vi "Details Display Dialog.vi"(0 "Source":string, 1 "Start":i32[](array[numeric]), 2 "Length":i32[](array[numeric]), 5 "Details":string="reason for problem", 7 "dialog type":T2, 9 "Error or Warning":bool, 11 "contname":string="Continue", 12 "stopname":string="Stop", 13 "okname":string="OK") -> (15 "stop event propagated":bool)   [LabVIEW 2011]
uses:
  DialogTypeEnum.ctl
  ErrWarn.ctl
  eventvkey.ctl
panel:
  in  "truncated message":string="(source truncated)"
  in  "truncated & CH message":string="(source truncated; see Context Help window)"
  out "Source of Error":string
  out "scrollbar text":string
  in  "Test for size":string
  out "text":string
  out "Error or Warning Glyph":T1=TRUE
  in  "OK":bool
  in  "Stop":bool
  in  "Continue":bool
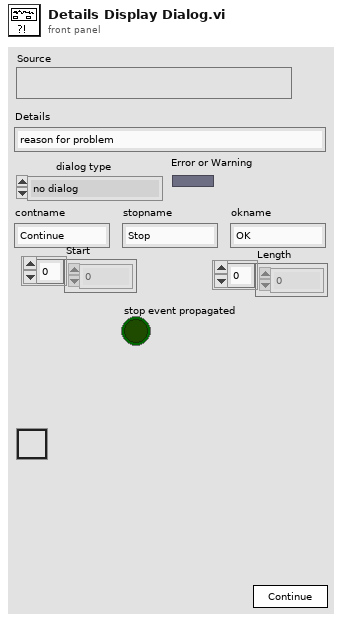
[diagram p1: front panel]
types:
  T1 = typedef "ErrWarn.ctl" = bool
  T2 = typedef "DialogTypeEnum.ctl" = enum16{"no dialog", "OK message", "continue or stop message", "auto error handling dialog", "OK message + warnings", "continue/stop + warnings"}
  T3 = typedef "eventvkey.ctl" = enum16{"ASCII", "Enter", "Return", "Shift", "Ctrl", "Alt", "Cmd", "Opt", "Caps", "NumLock", "Clear", "Break", "Up", "Down", "Left", "Right", "Insert", "Delete", "Home", "End", "PageUp", "PageDown", "Escape", "Help", "Pause", "ScrollLock", "F1", "F2", "F3", "F4", "F5", "F6", "F7", "F8", "F9", "F10", "F11", "F12", "F13", "F14", "F15", "F16", "F17", "F18", "F19", "F20", "F21", "F22", "F23", "F24", "Play", "VolumeUp", "VolumeDown", "Mute", "Two Byte Char"}
  T4 = typedef "LVRectTypeDef.ctl" = cluster{"left":i16, "top":i16, "right":i16, "bottom":i16}
  T5 = cluster{"Control":bool, "Shift":bool, "Key":string}
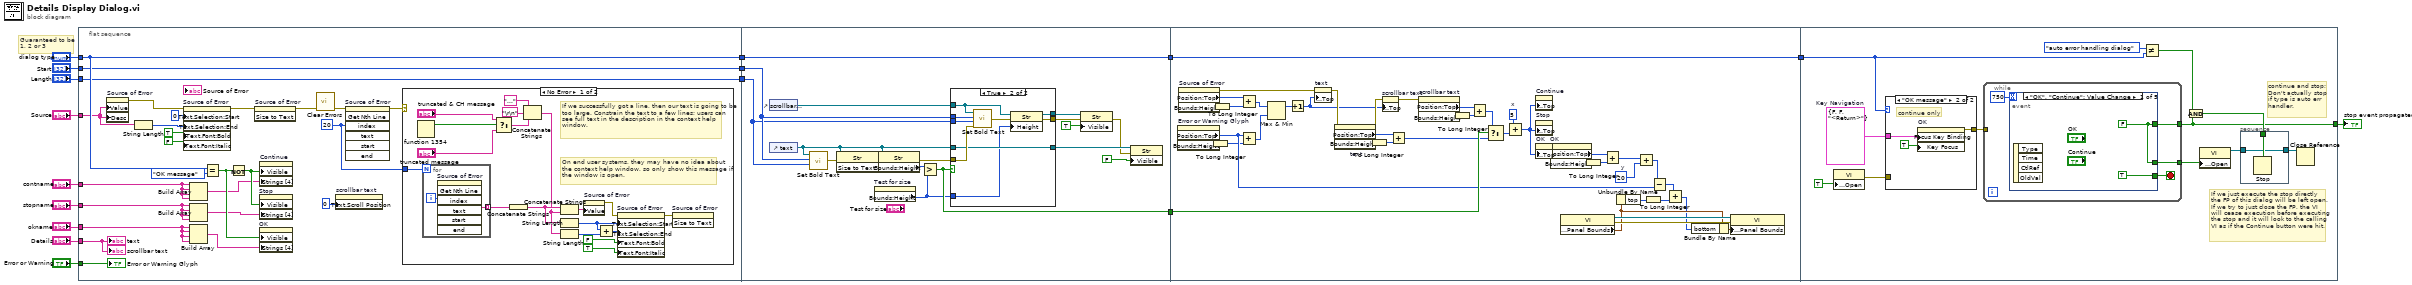
[diagram p0: block diagram]
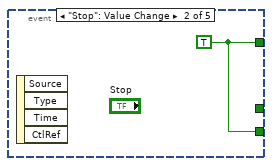
[diagram p4: hidden frame]
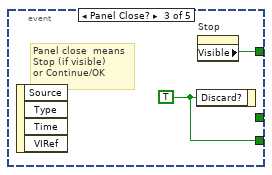
[diagram p5: hidden frame]
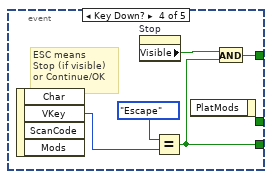
[diagram p6: hidden frame]
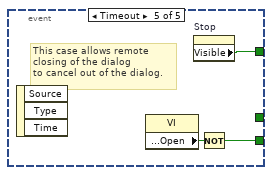
[diagram p7: hidden frame]
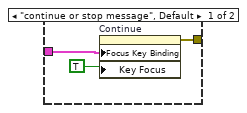
[diagram p8: hidden frame]
diagram:
  # "Guaranteed to be\n1, 2 or 3"
  n1 = flat-sequence {
    tunnel: [w25] -> w15
    tunnel: "dialog type" -> [w25]
    tunnel: "contname" -> [w24]
    tunnel: "stopname" -> [w23]
    tunnel: "okname" -> [w22]
    tunnel: "Source" -> [w17]
    tunnel: "Details" -> [w21]
    tunnel: "Error or Warning" -> [w20]
    tunnel: [w19] -> w4
    tunnel: [w18] -> w3
    tunnel: "Start" -> [w19]
    tunnel: "Length" -> [w18]
    tunnel: w15 -> [w65]
    tunnel: [w65] -> w14
    tunnel: [w71] -> w13
    tunnel: w4 -> [w64]
    tunnel: w3 -> [w63]
    tunnel: w14 -> [w98]
    tunnel: [w98] -> w12
    tunnel: w13 -> [w133]
    tunnel: [w134] -> w16
    tunnel: w12 -> [w136]
    frame #0 {
      w32 = u32 20 ("index")
      n2 = property on="Source of Error" class="Str"("Value"=w17, "Desc"=w17) -> (error out=w31:errorcluster)  [unwired: 2 in, 1 out]
      n3 = String Length(string=w17) -> (length=w28:i32)
      n4 = property on="Source of Error" class="Str"(error in=w31, "Text.Selection:Start"=u32 0, "Text.Selection:End"=w28, "Text.Font:Bold"=TRUE, "Text.Font:Italic"=FALSE) -> (error out=w30:errorcluster)  [unwired: 1 in, 1 out]
      n5 = Build Array(w24, w24, w24, w24) -> (w40:string[])
      n6 = Build Array(w23, w23, w23, w23) -> (w39:string[])
      n7 = Build Array(w22, w22, w22, w22) -> (w38:string[])
      n8 = Equal?(x=w25, y=DialogTypeEnum."OK message" ("dialog type")) -> (x = y?=w42:bool)
      n9 = Not(x=w42) -> (.not. x?=w41:bool)
      n10 = invoke on="Source of Error" class="Str" method="Size to Text"(error in=w30) -> (error out=w35:errorcluster)  [unwired: 2 in, 2 out]
      n11 = property on="Continue" class="Bool"("Visible"=w41, "Strings [4]"=w40) -> ()  [unwired: 2 in, 2 out]
      n12 = property on="Stop" class="Bool"("Visible"=w41, "Strings [4]"=w39) -> ()  [unwired: 2 in, 2 out]
      n13 = property on="OK" class="Bool"("Visible"=w42, "Strings [4]"=w38) -> ()  [unwired: 2 in, 2 out]
      n14 = call "Clear Errors.vi"("error in (no error)"=w35) -> ("error out"=w34:errorcluster)  [unwired: 6 in]
      n15 = property on="scrollbar text" class="Str"("Text.Scroll Position"=u32 0) -> ()  [unwired: 2 in, 2 out]
      n16 = invoke on="Source of Error" class="Str" method="Get Nth Line"(error in=w34, "index"=w32) -> (error out=w33:errorcluster)  [unwired: 5 in, 6 out]
      n17 = case shown="No Error" w33 {
        tunnel: w32 -> [w60 _]
        frame No Error {
          # "If we successfully got a line, then our text is going to be too large. Constrain the text to a few lines; users can see full text in the description in the context help window."
          # "On end user systems, they may have no idea about\nthe context help window, so only show this message if\nthe window is open."
          n18 = fn#1354() -> (1:w50:bool)  [unwired: 1 out]
          n19 = for {
            N: w60 -> [_]
            tunnel: [w61] -> w58 mode=indexing
            i -> [w62]
            n20 = invoke on="Source of Error" class="Str" method="Get Nth Line"("index"=w62) -> ("text"=w61:string)  [unwired: 6 in, 6 out]
          }
          n21 = Select(t="truncated & CH message", s=w50, f="truncated message") -> (s? t:f=w47:string)
          n22 = Concatenate Strings(w58) -> (w57:string)
          n23 = Concatenate Strings("..." ("string"), "\r\n", w47) -> (w44:string)
          n24 = Concatenate Strings(w57, w44) -> (w59:string)
          n25 = String Length(string=w57) -> (length=w52:i32)
          n26 = String Length(string=w44) -> (length=w49:i32)
          n27 = property on="Source of Error" class="Str"("Value"=w59) -> (error out=w54:errorcluster)  [unwired: 2 in, 1 out]
          n28 = Add(x=w52, y=w49) -> (x+y=w51:i32)
          n29 = property on="Source of Error" class="Str"(error in=w54, "Text.Selection:Start"=w52, "Text.Selection:End"=w51, "Text.Font:Bold"=FALSE, "Text.Font:Italic"=TRUE) -> (error out=w53:errorcluster)  [unwired: 1 in, 1 out]
          n30 = invoke on="Source of Error" class="Str" method="Size to Text"(error in=w53) -> ()  [unwired: 2 in, 3 out]
        }
        frame Error {
          # "An error at this point means that there is no line to fetch. That's good. We do not want the text getting too large."
        }
      }
      "Error or Warning Glyph" <- w20
      "scrollbar text" <- w21
      "text" <- w21
    }
    frame #1 {
      n31 = control-ref of="scrollbar text"() -> (w74:refnum<vi>)
      n32 = control-ref of="text"() -> (w66:refnum<vi>)
      n33 = call "Set Bold Text.vi"("Length"=w63, "Start"=w64, "text"=w66) -> ("error out"=w69:errorcluster)  [unwired: 3 in]
      n34 = invoke class="Str" method="Size to Text"(reference=w66, error in=w69) -> (error out=w70:errorcluster)  [unwired: 1 in, 2 out]
      n35 = property on="Test for size" class="Str"() -> ("Bounds:Height"=w68:u32)  [unwired: 2 in, 2 out]
      n36 = property class="Str"(reference=w66, error in=w70) -> (error out=w78:errorcluster, "Bounds:Height"=w79:u32)  [unwired: 1 out]
      n37 = Greater?(x=w79, y=w68) -> (0:w71:bool)
      n38 = case shown="True" w71 {
        tunnel: w78 -> [w82 w91]
        tunnel: w64 -> [_ w90]
        tunnel: w63 -> [_ w89]
        tunnel: [w82 w86] -> w67
        tunnel: w66 -> [w81 w88]
        tunnel: [w81 w83] -> w76
        tunnel: [w80 w88] -> w75
        tunnel: w74 -> [w80 w84]
        tunnel: w68 -> [_ w87]
        frame False {
        }
        frame True {
          n39 = call "Set Bold Text.vi"("error in"=w91, "Length"=w89, "Start"=w90, "text"=w84) -> ("error out"=w85:errorcluster)  [unwired: 2 in]
          n40 = property class="Str"(reference=w84, error in=w85, "Height"=w87) -> (reference out=w83:refnum<vi>, error out=w86:errorcluster)
        }
      }
      n41 = property class="Str"(reference=w76, error in=w67, "Visible"=TRUE ("Defer Panel Updates")) -> (error out=w72:errorcluster)  [unwired: 1 out]
      n42 = property class="Str"(reference=w75, error in=w72, "Visible"=FALSE ("Defer Panel Updates")) -> ()  [unwired: 2 out]
    }
    frame #2 {
      w119 = 20  # y
      w124 = 5  # x
      n43 = property on="Error or Warning Glyph" class="Bool"() -> ("Position:Top"=w114:i32, "Bounds:Height"=w130:u32)  [unwired: 2 in, 2 out]
      n44 = property on="Source of Error" class="Str"() -> (error out=w99:errorcluster, "Position:Top"=w101:i32, "Bounds:Height"=w100:u32)  [unwired: 2 in, 1 out]
      n45 = To Long Integer(number=w130) -> (32bit integer=w97:i32)
      n46 = To Long Integer(number=w100) -> (32bit integer=w96:i32)
      n47 = Add(x=w101, y=w96) -> (x+y=w132:i32)
      n48 = Add(x=w114, y=w97) -> (x+y=w131:i32)
      n49 = Max & Min(x=w132, y=w131) -> (max(x,y)=w129:i32)  [unwired: 1 out]
      n50 = Increment(x=w129) -> (x+1=w107:i32)
      n51 = property on="text" class="Str"(error in=w99, "Position:Top"=w107) -> (error out=w109:errorcluster)  [unwired: 1 in, 1 out]
      n52 = property on="text" class="Str"(error in=w109) -> (error out=w108:errorcluster, "Position:Top"=w106:i32, "Bounds:Height"=w105:u32)  [unwired: 1 in, 1 out]
      n53 = To Long Integer(number=w105) -> (32bit integer=w95:i32)
      n54 = property on="scrollbar text" class="Str"(error in=w108, "Position:Top"=w107) -> (error out=w128:errorcluster)  [unwired: 1 in, 1 out]
      n55 = Add(x=w106, y=w95) -> (x+y=w103:i32)
      n56 = property on="scrollbar text" class="Str"(error in=w128) -> ("Position:Top"=w127:i32, "Bounds:Height"=w126:u32)  [unwired: 1 in, 2 out]
      n57 = To Long Integer(number=w126) -> (32bit integer=w94:i32)
      n58 = Add(x=w127, y=w94) -> (x+y=w104:i32)
      n59 = Select(t=w104, s=w133, f=w103) -> (s? t:f=w102:i32)
      n60 = Add(x=w124, y=w102) -> (x+y=w125:i32)
      n61 = property on="Continue" class="Bool"("Position:Top"=w125) -> ()  [unwired: 2 in, 2 out]
      n62 = property on="Stop" class="Bool"("Position:Top"=w125) -> ()  [unwired: 2 in, 2 out]
      n63 = property on="OK" class="Bool"("Position:Top"=w125) -> (error out=w123:errorcluster)  [unwired: 2 in, 1 out]
      n64 = property on="OK" class="Bool"(error in=w123) -> ("Position:Top"=w121:i32, "Bounds:Height"=w122:u32)  [unwired: 1 in, 2 out]
      n65 = property class="VI"() -> (reference out=w116:refnum<vi>, error out=w117:errorcluster, "Front Panel Window:Panel Bounds"=w113:T4)  [unwired: 2 in]
      n66 = To Long Integer(number=w122) -> (32bit integer=w93:i32)
      n67 = Add(x=w121, y=w93) -> (x+y=w120:i32)
      n68 = Unbundle By Name(w113) -> ("top"=w111:i16)
      n69 = Add(x=w120, y=w119) -> (x+y=w115:i32)
      n70 = To Long Integer(number=w111) -> (32bit integer=w92:i32)
      n71 = Subtract(x=w115, y=w114) -> (x-y=w112:i32)
      n72 = Add(x=w112, y=w92) -> (x+y=w110:i32)
      n73 = Bundle By Name(cluster=w113, "bottom"=w110) -> (w118:T4)
      n74 = property class="VI"(reference=w116, error in=w117, "Front Panel Window:Panel Bounds"=w118) -> ()  [unwired: 2 out]
    }
    frame #3 {
      w145 = T5 {"Control"=FALSE, "Shift"=FALSE, "Key"="<Return>"}  # Key Navigation
      # "If we just execute the stop directly\nthe FP of this dialog will be left open.\nIf we try to just close the FP, the VI\nwill cease execution before executing\nthe stop and it will look to the calling\nVI as if the Continue button were hit."
      # "continue and stop;\nDon't actually stop\nif type is auto err\nhandler."
      n75 = property class="VI"("Front Panel Window:Open"=TRUE) -> (error out=w144:errorcluster)  [unwired: 2 in, 1 out]
      n76 = case shown="\"OK message\"" w136 {
        tunnel: w145 -> [w167 w170]
        tunnel: w144 -> [_ _]
        tunnel: [w165 w168] -> w142
        frame "continue or stop message", Default {
          n77 = property on="Continue" class="Bool"("Focus Key Binding"=w167, "Key Focus"=TRUE) -> (error out=w165:errorcluster)  [unwired: 2 in, 1 out]
        }
        frame "OK message" {
          # "continue only"
          n78 = property on="OK" class="Bool"("Focus Key Binding"=w170, "Key Focus"=TRUE) -> (error out=w168:errorcluster)  [unwired: 2 in, 1 out]
        }
      }
      n79 = while {
        tunnel: w142 -> [_]
        tunnel: [w150] -> w134
        tunnel: [w149] -> w135
        stop <- w151 stop-if-true
        n80 = event shown="[0] \"OK\", \"Continue\": Value Change" {
          selector: _ -> [_ _ _ _ _]
          dyn-events: _ -> [_ _ _ _ _]
          timeout: 750 -> [_ _ _ _ _]
          tunnel: [TRUE ("Stop") w154 w156 w157 w162] -> w151
          tunnel: [w153 w154 w155 w160 w164] -> w150
          tunnel: [w153 _ _ _ _] -> w149
          event "OK", "Continue": Value Change {
            w153 = FALSE ("Stop")
            n81 = event-data() -> ()  [unwired: 1 in, 4 out]
          }
          event "Stop": Value Change {
            w154 = TRUE
            n82 = event-data() -> ()  [unwired: 1 in, 4 out]
          }
          event Panel Close? {
            w156 = TRUE ("Discard?")
            # "Panel close  means\nStop (if visible)\nor Continue/OK"
            n83 = event-data() -> ()  [unwired: 1 in, 4 out]
            n84 = event-data("Discard?"=w156) -> ()  [unwired: 1 in, 1 out]
            n85 = property on="Stop" class="Bool"() -> ("Visible"=w155:bool)  [unwired: 2 in, 2 out]
          }
          event Key Down? {
            # "ESC means\nStop (if visible)\nor Continue/OK"
            n86 = event-data() -> ("VKey"=w159:T3)  [unwired: 1 in, 3 out]
            n87 = property on="Stop" class="Bool"() -> ("Visible"=w161:bool)  [unwired: 2 in, 2 out]
            n88 = Equal?(x=eventvkey."Escape", y=w159) -> (x = y?=w157:bool)
            n89 = event-data() -> ()  [unwired: 2 in, 1 out]
            n90 = And(x=w161, y=w157) -> (x .and. y?=w160:bool)
          }
          event Timeout {
            # "This case allows remote\nclosing of the dialog\nto cancel out of the dialog."
            n91 = event-data() -> ()  [unwired: 1 in, 3 out]
            n92 = property class="VI"() -> ("Front Panel Window:Open"=w163:bool)  [unwired: 2 in, 2 out]
            n93 = property on="Stop" class="Bool"() -> ("Visible"=w164:bool)  [unwired: 2 in, 2 out]
            n94 = Not(x=w163) -> (.not. x?=w162:bool)
          }
        }
      }
      n95 = Not Equal?(x=DialogTypeEnum."auto error handling dialog" ("dialog type"), y=w136) -> (x != y?=w141:bool)
      n96 = And(x=w141, y=w134) -> (x .and. y?=w140:bool)
      n97 = property class="VI"("Front Panel Window:Open"=w135) -> (reference out=w138:refnum<vi>)  [unwired: 2 in, 1 out]
      n98 = stacked-sequence {
        tunnel: w138 -> [w146]
        tunnel: w140 -> [w147]
        tunnel: [w146] -> w139
        frame #0 {
          n99 = Stop(stop? (T)=w147) -> ()
        }
      }
      n100 = Close Reference(reference=w139) -> ()  [unwired: 1 in, 1 out]
    }
  }
  "stop event propagated" <- w16
